vi "RoboTaxi VI_Wifi.vi"() -> ()   [LabVIEW 2022 SP3]
doc: "This example performs writes and reads on a serial port, as directed by the user. You can press the Write and Read buttons, and change the Read Count, while the example is running.\n\nThe parameters set for the serial port must match the parameters of the connected instrument or device. In this example, the Read Count parameter specifies the number of bytes that the serial port reads. If there were more bytes at the port than the specified number, those bytes would not be read. If there were less bytes at the port than the specified number, you would receive a timeout error.\n\nThis example expands upon the flow control options for XON and XOFF, allowing the user to choose those control characters. Also, the user can enable or disable a termination character. Some devices require a termination character in order to identify the end of command strings. Some devices send a termination character to signify the end of data to be read. This example shows how you can end the Read operation once a termination character is detected in the buffer and/or append a termination character at the end of the Write data."
uses:
  ESP32-PSOC-State Machine.ctl
panel:
  in  "address":string="10.0.0.127"
  in  "Stop Driving":bool
  in  "Right":bool
  in  "Left":bool
  in  "Backward":bool
  in  "Forward":bool
  in  "Manual":bool
  in  "Autonomous":bool
  in  "Track 2":bool
  in  "Track 1":bool
  out "error":bool
  out "Response 2":string
  in  "Toggle LED":bool
  in  "Enum":T1
  in  "Stop":bool
  out "Read Count":u32=1000
  out "Response":string
  # "ESP32 Control"
  # "Track Selection"
  # "Driving Mode"
  # "Manual Override"
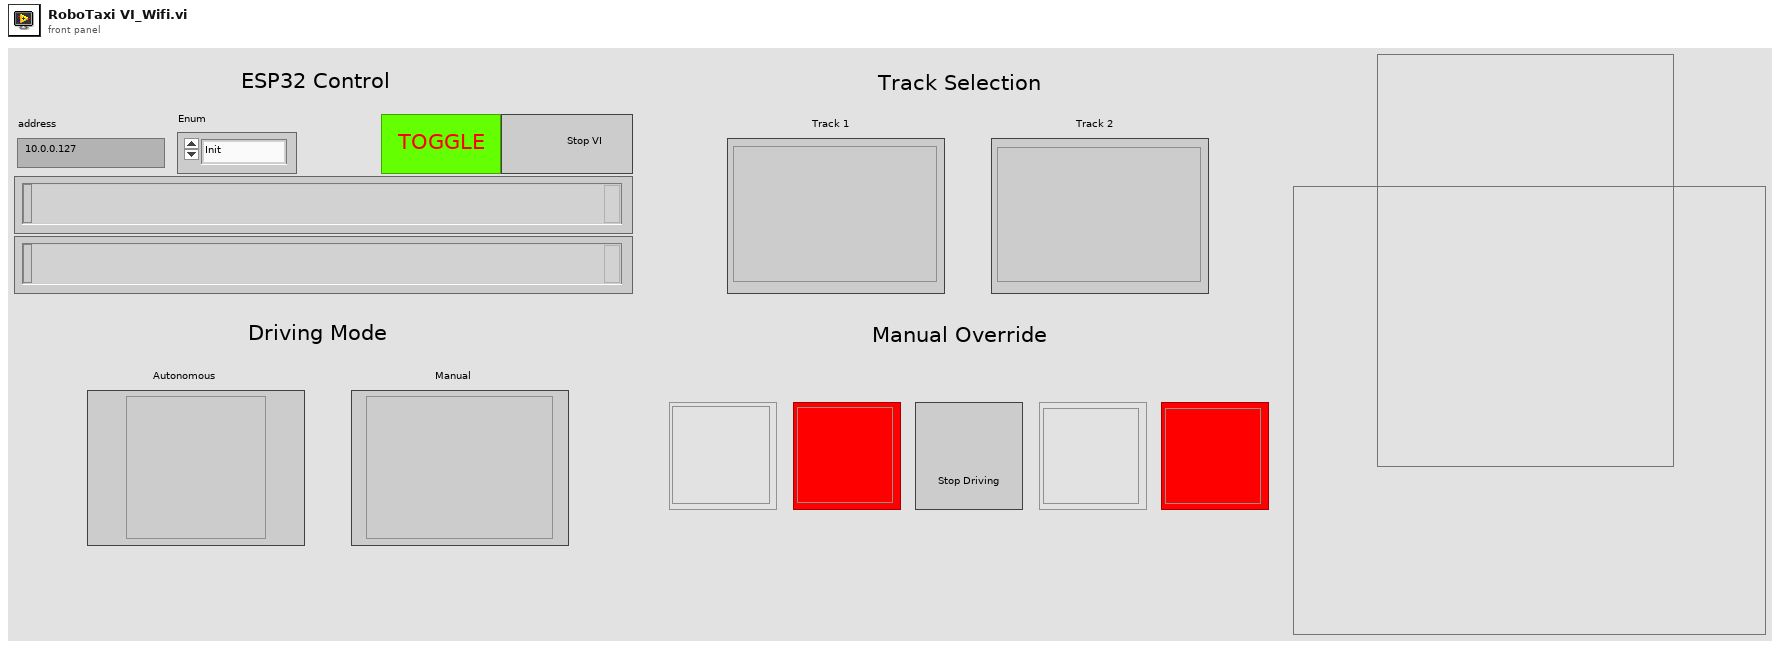
[diagram p1: front panel]
types:
  T1 = typedef "ESP32-PSOC-State Machine.ctl" = enum8{"Init", "Connect", "idle", "send", "wait", "receive", "que", "error", "exit"}
  T2 = enum16{"Standard", "Buffered", "CRLF", "Immediate"}
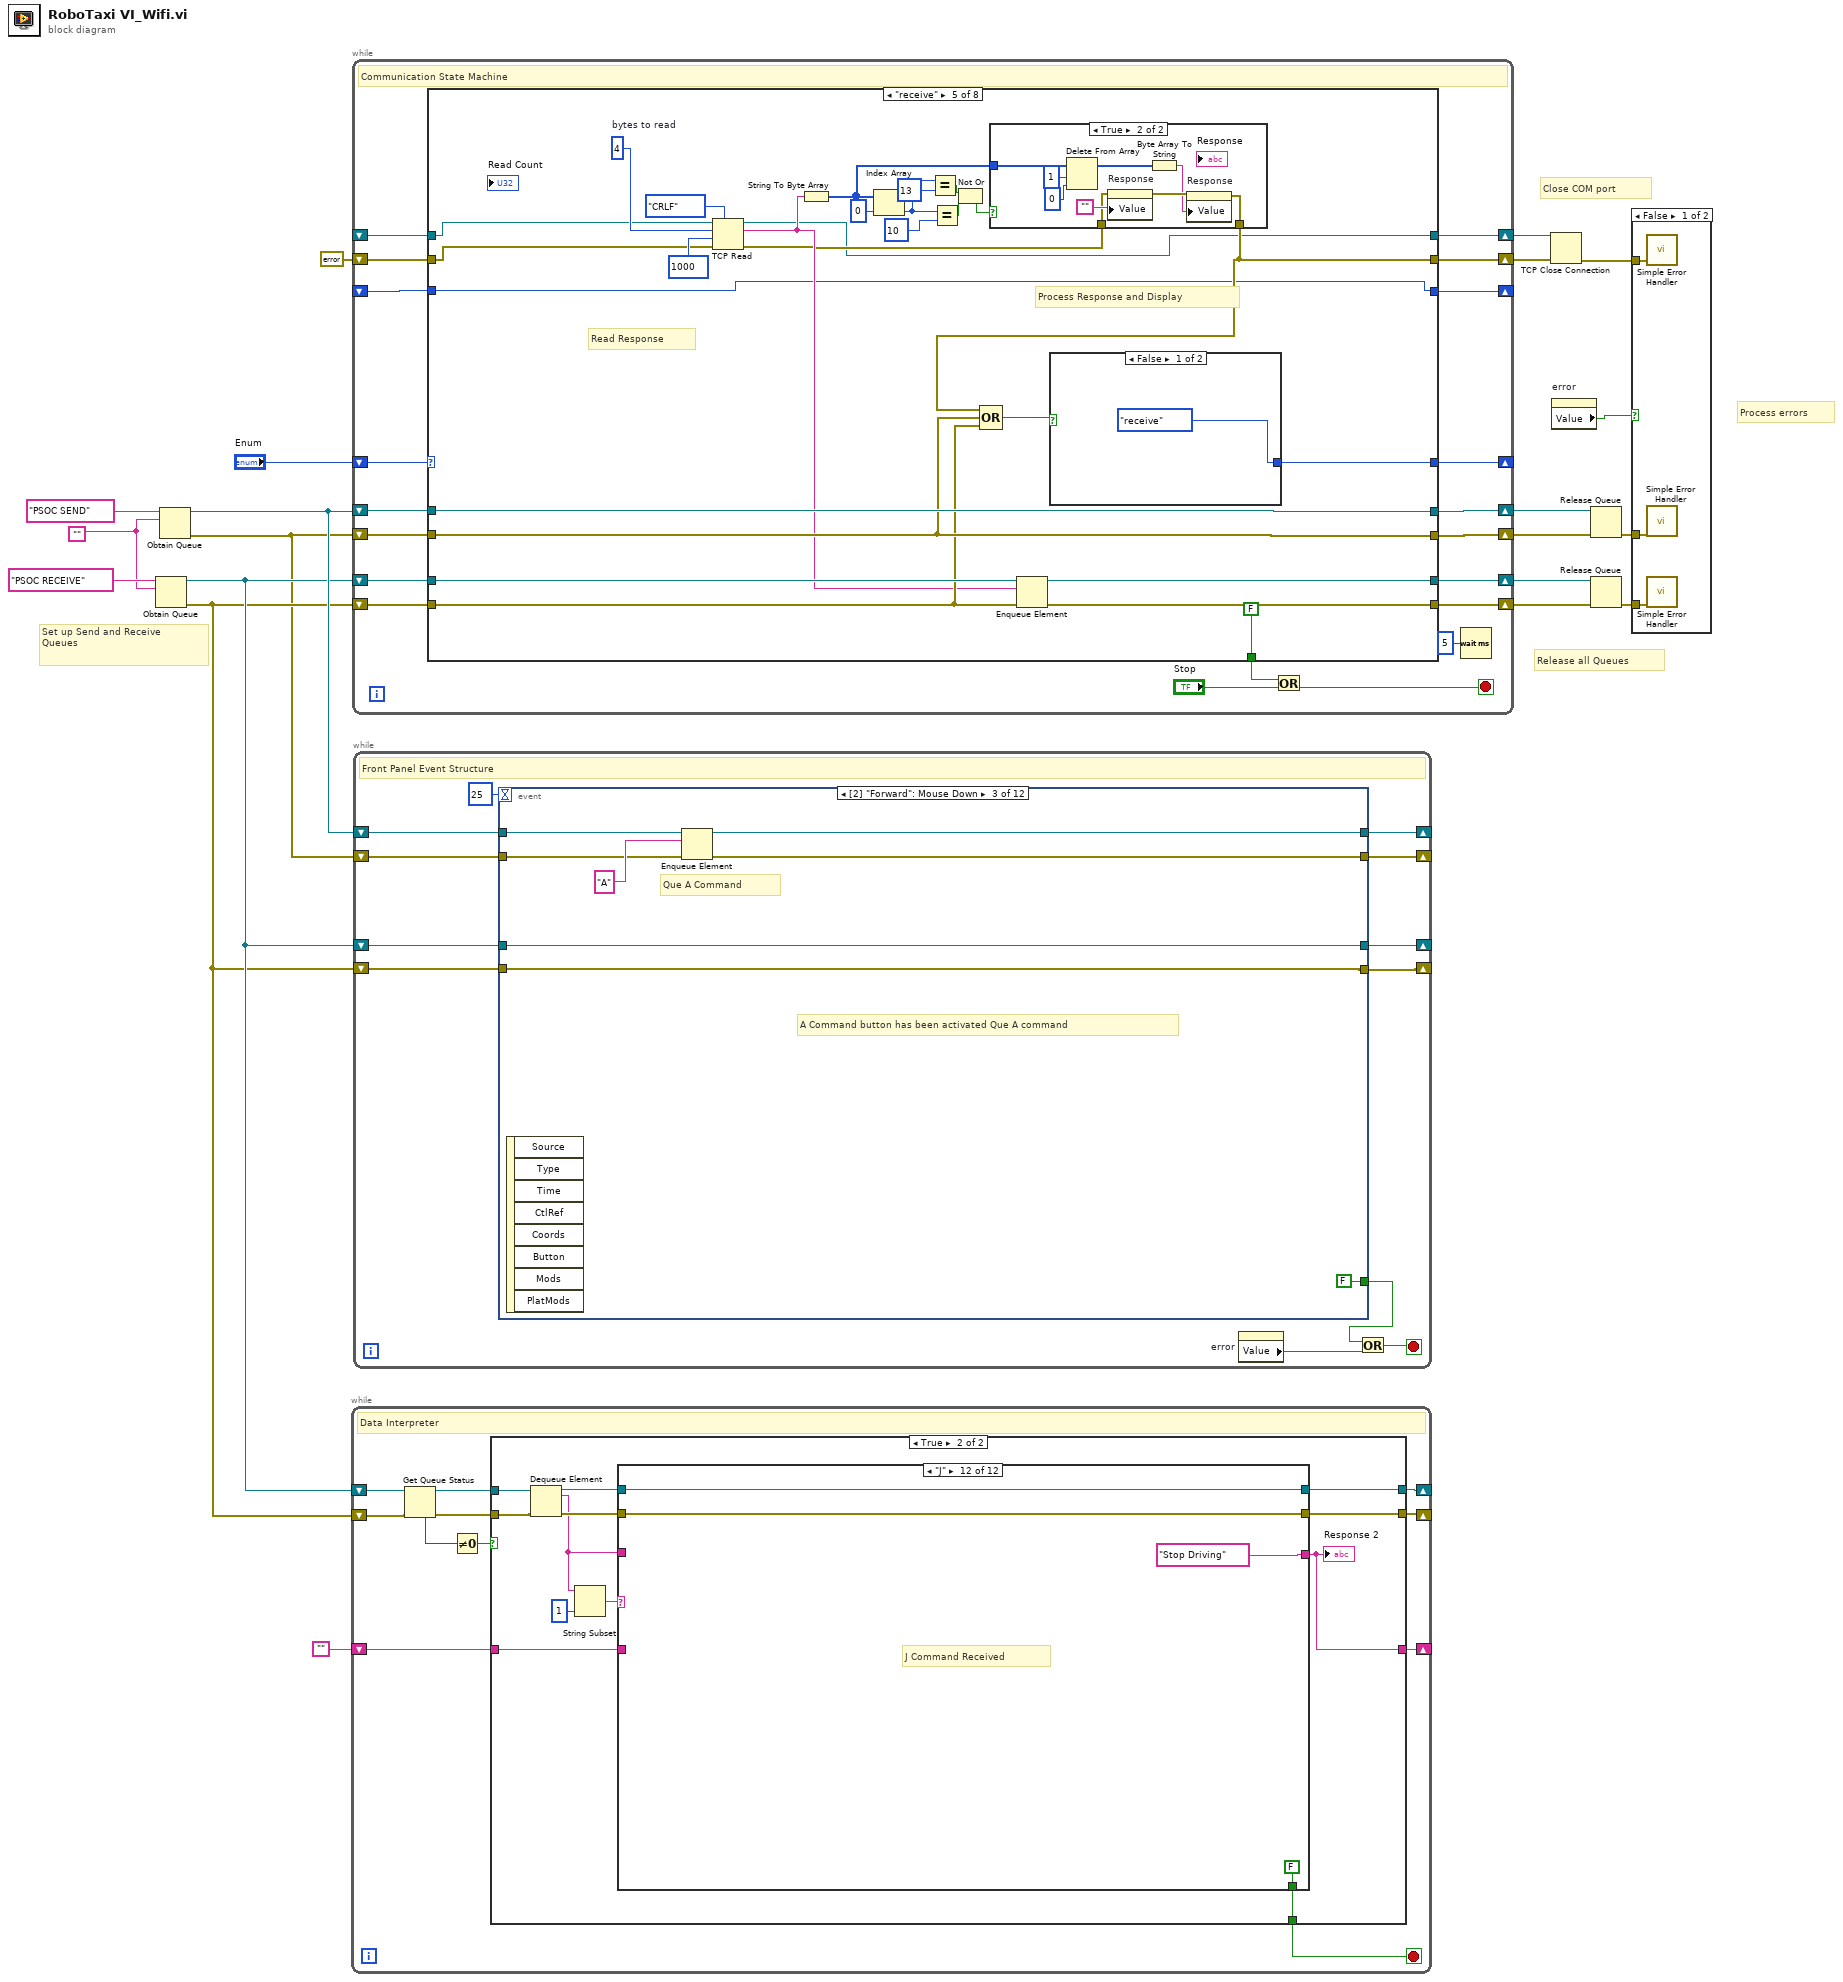
[diagram p0: block diagram]
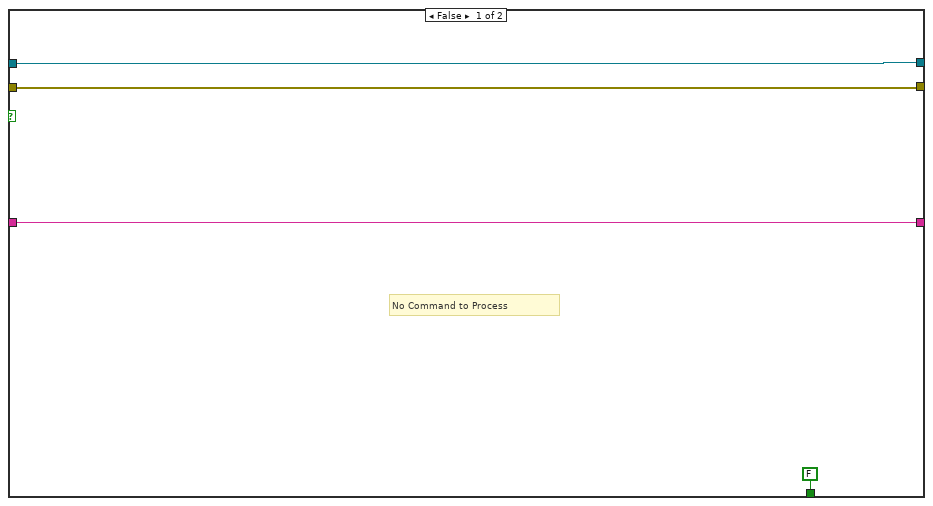
[diagram p3: hidden frame]
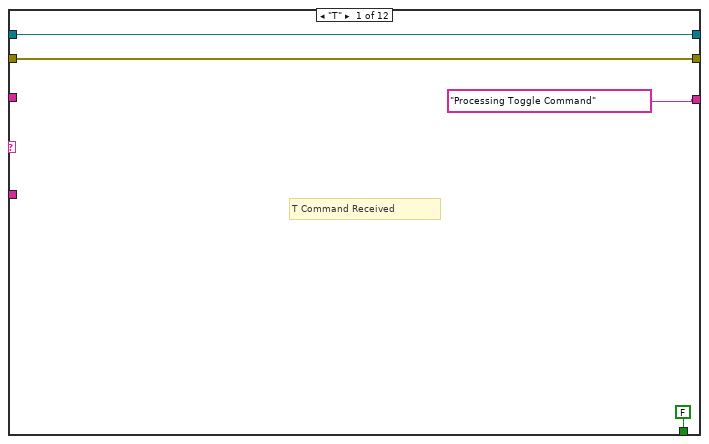
[diagram p4: hidden frame]
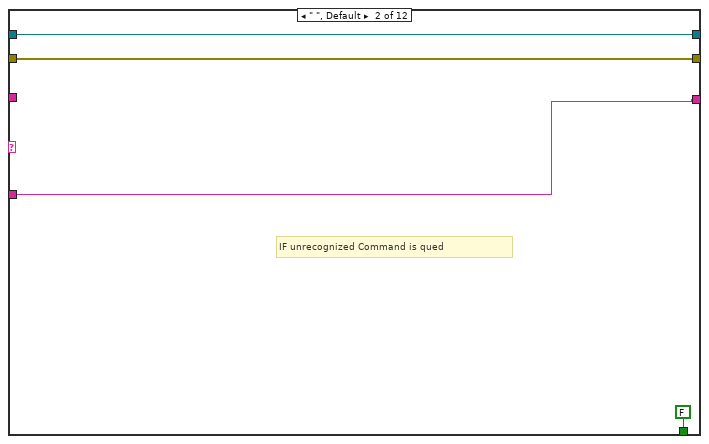
[diagram p5: hidden frame]
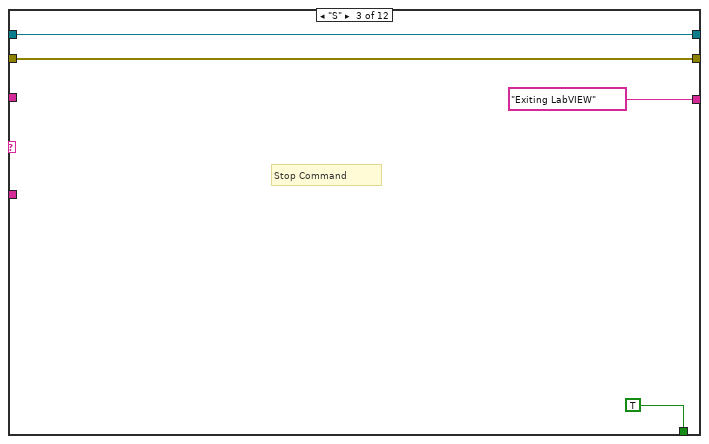
[diagram p6: hidden frame]
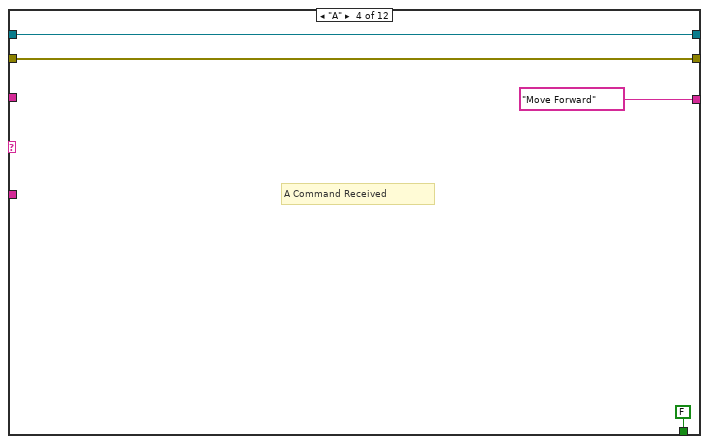
[diagram p7: hidden frame]
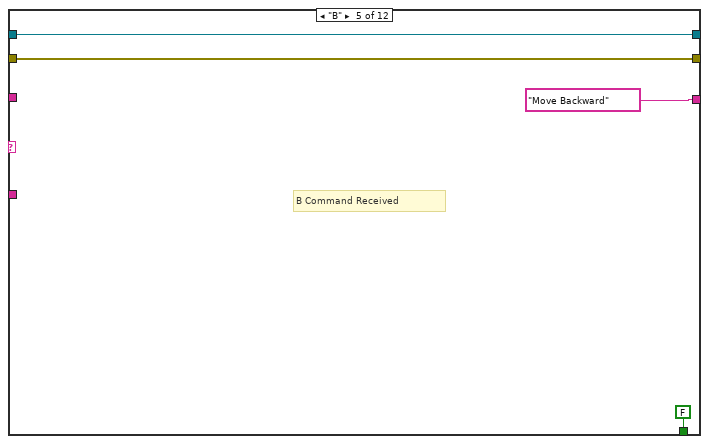
[diagram p8: hidden frame]
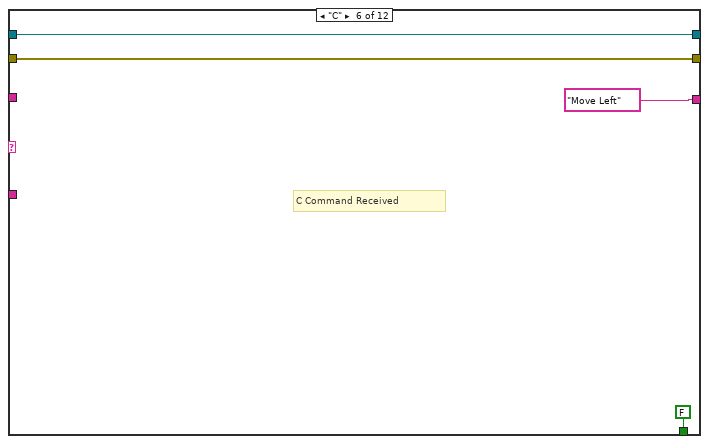
[diagram p9: hidden frame]
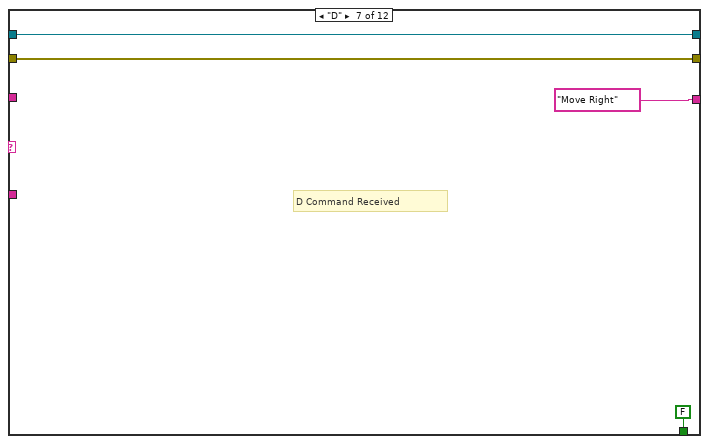
[diagram p10: hidden frame]
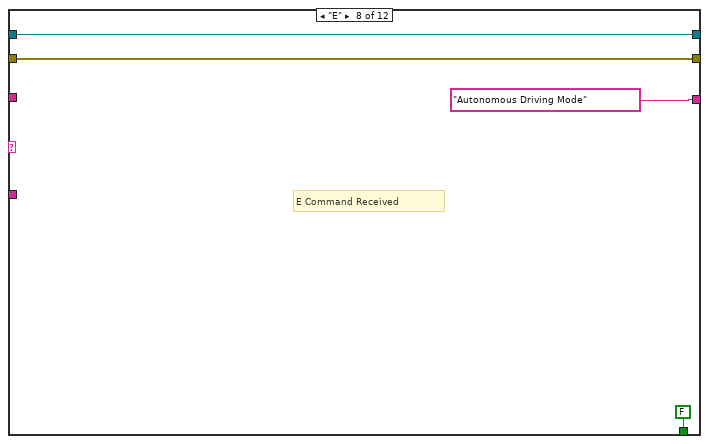
[diagram p11: hidden frame]
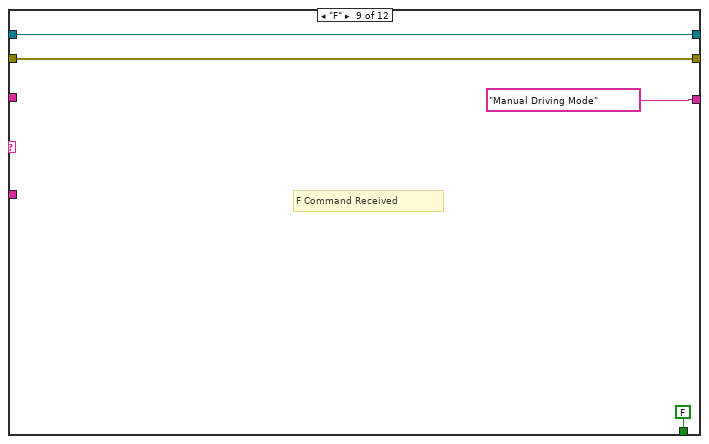
[diagram p12: hidden frame]
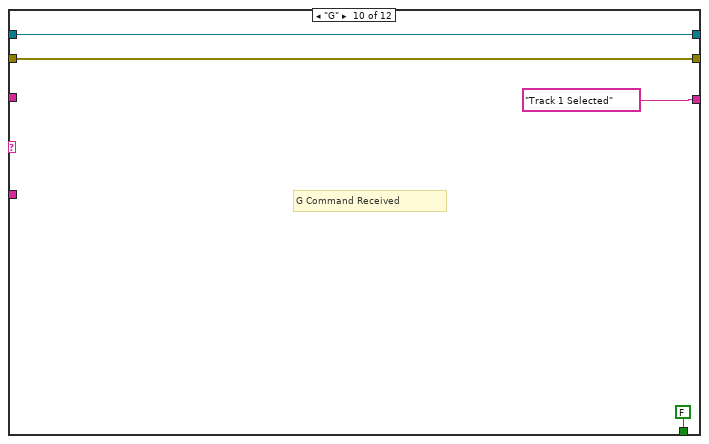
[diagram p13: hidden frame]
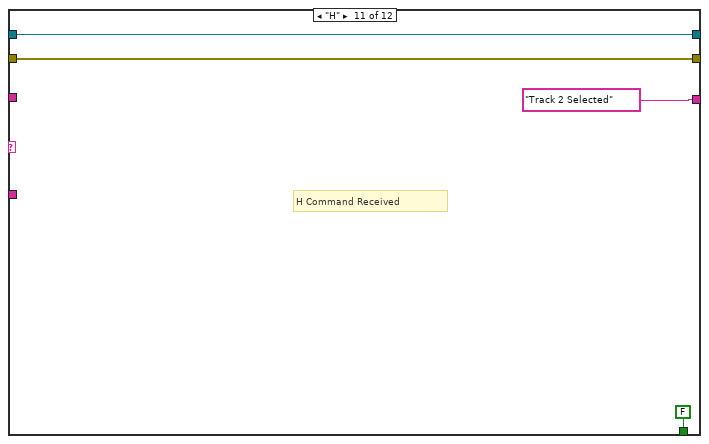
[diagram p14: hidden frame]
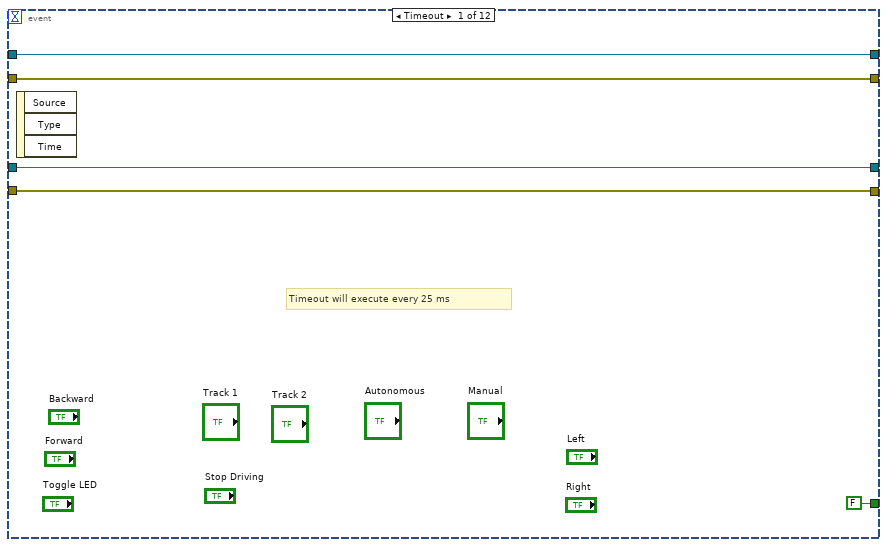
[diagram p15: hidden frame]
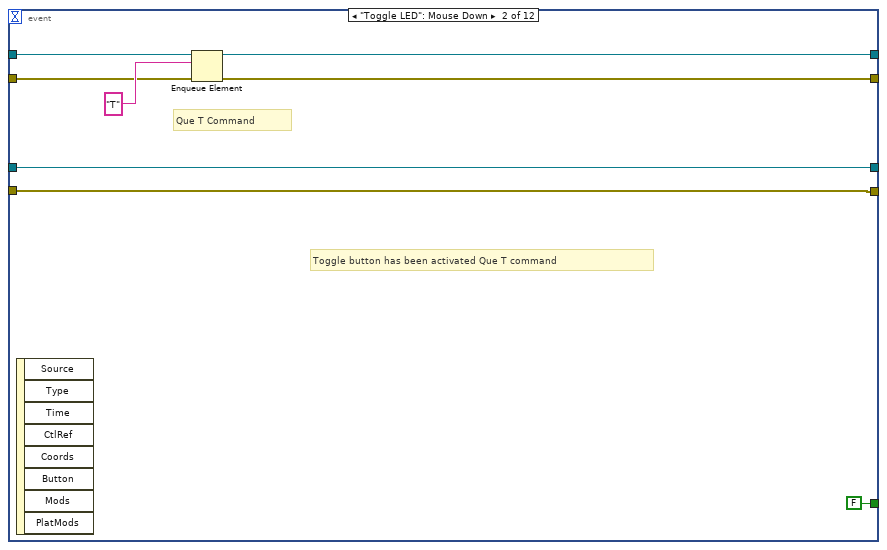
[diagram p16: hidden frame]
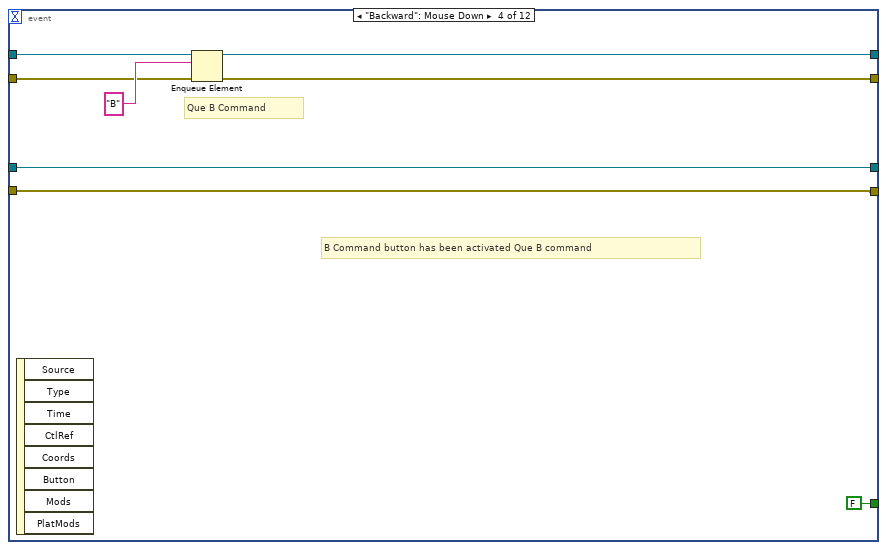
[diagram p17: hidden frame]
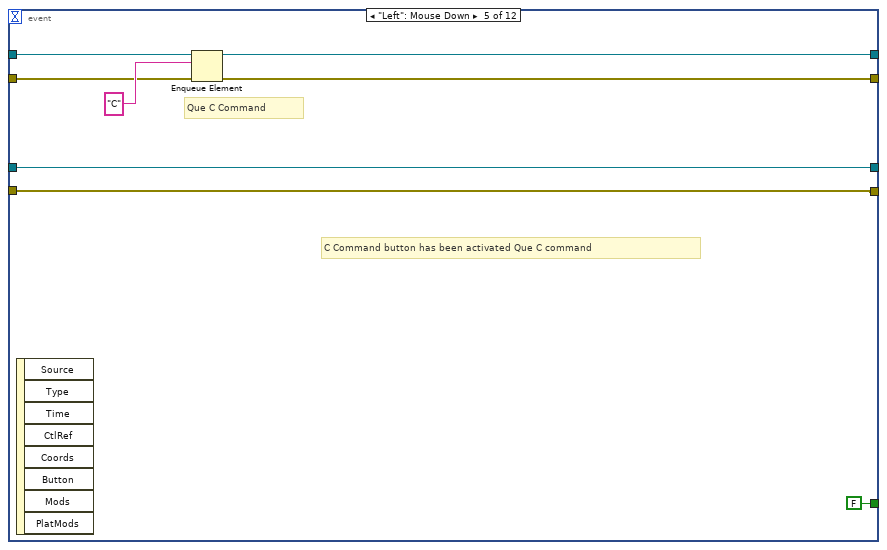
[diagram p18: hidden frame]
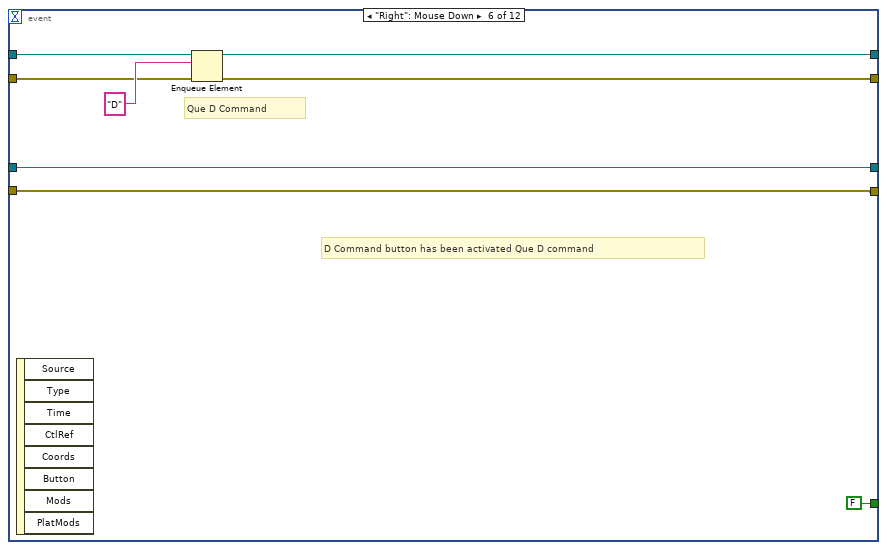
[diagram p19: hidden frame]
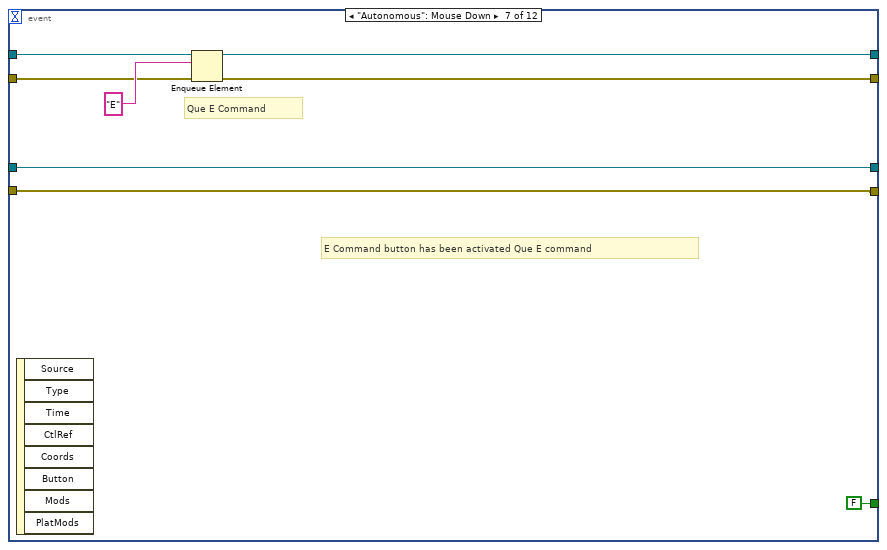
[diagram p20: hidden frame]
diagram:
  w12 = ""
  # "Process errors"
  # "Release all Queues"
  # "Close COM port"
  # "Set up Send and Receive\nQueues"
  n1 = Obtain Queue(name (unnamed)="PSOC RECEIVE", element data type=w12) -> (queue out=w11:refnum<queue>, error out=w10:errorcluster)  [unwired: 3 in, 1 out]
  n2 = Obtain Queue(name (unnamed)="PSOC SEND", element data type=w12) -> (queue out=w14:refnum<queue>, error out=w5:errorcluster)  [unwired: 3 in, 1 out]
  n3 = while {
    shift-right: [w25] -> _
    shift-left: w11 -> [w31]
    shift-right: [w24] -> _
    shift-left: w10 -> [w30]
    shift-right: [w22] -> _
    shift-left: "" -> [w21]
    stop <- w23 stop-if-true
    # "Data Interpreter"
    n4 = Get Queue Status(queue=w31, error in (no error)=w30) -> (queue out=w27:refnum<queue>, error out=w26:errorcluster, # elements in queue=w29:i32)  [unwired: 1 in, 5 out]
    n5 = Not Equal To 0?(x=w29) -> (x != 0?=w28:bool)
    n6 = case shown="True" w28 {
      tunnel: w27 -> [w35 w47]
      tunnel: w26 -> [w34 w46]
      tunnel: [w35 w41] -> w25
      tunnel: [w34 w40] -> w24
      tunnel: [FALSE w39] -> w23
      tunnel: [w32 w37] -> w22
      tunnel: w21 -> [w32 w36]
      frame False {
        # "No Command to Process"
      }
      frame True {
        n7 = Dequeue Element(queue=w47, error in (no error)=w46) -> (queue out=w45:refnum<queue>, element=w38:string, error out=w44:errorcluster)  [unwired: 1 in, 1 out]
        n8 = String Subset(string=w38, length (rest)=1 ("length (rest)")) -> (substring=w42:string)  [unwired: 1 in]
        n9 = case shown="\"J\"" w42 {
          tunnel: w45 -> [w51 w55 w59 w63 w67 w71 w75 w79 w83 w87 w91 w95]
          tunnel: w44 -> [w50 w54 w58 w62 w66 w70 w74 w78 w82 w86 w90 w94]
          tunnel: [w51 w55 w59 w63 w67 w71 w75 w79 w83 w87 w91 w95] -> w41
          tunnel: [w50 w54 w58 w62 w66 w70 w74 w78 w82 w86 w90 w94] -> w40
          tunnel: w38 -> [_ _ _ _ _ _ _ _ _ _ _ _]
          tunnel: [FALSE FALSE TRUE FALSE FALSE FALSE FALSE FALSE FALSE FALSE FALSE FALSE] -> w39
          tunnel: ["Processing Toggle Command" w52 "Exiting LabVIEW" "Move Forward" "Move Backward" "Move Left" "Move Right" "Autonomous Driving Mode" "Manual Driving Mode" "Track 1 Selected" "Track 2 Selected" "Stop Driving"] -> w37
          tunnel: w36 -> [_ w52 _ _ _ _ _ _ _ _ _ _]
          frame "T" {
            # "T Command Received"
          }
          frame " ", Default {
            # "IF unrecognized Command is qued"
          }
          frame "S" {
            # "Stop Command"
          }
          frame "A" {
            # "A Command Received"
          }
          frame "B" {
            # "B Command Received"
          }
          frame "C" {
            # "C Command Received"
          }
          frame "D" {
            # "D Command Received"
          }
          frame "E" {
            # "E Command Received"
          }
          frame "F" {
            # "F Command Received"
          }
          frame "G" {
            # "G Command Received"
          }
          frame "H" {
            # "H Command Received"
          }
          frame "J" {
            # "J Command Received"
          }
        }
        "Response 2" <- w37
      }
    }
  }
  n10 = while {
    shift-right: [w107] -> w20
    shift-left: w14 -> [w115]
    shift-right: [w106] -> w18
    shift-left: w5 -> [w114]
    shift-right: [w105] -> w19
    shift-left: w11 -> [w113]
    shift-right: [w104] -> w15
    shift-left: w10 -> [w112]
    shift-right: [w99] -> _
    shift-left: "Enum" -> [w98]
    shift-right: [w111] -> w3
    shift-left: _ -> [w108]
    shift-right: [w110] -> w2
    shift-left: errorcluster {"status"=FALSE, "code"=0, "source"=""} ("error out") -> [w109]
    shift-right: [w103] -> _
    shift-left: _ -> [w102]
    stop <- w97 stop-if-true
    # "Communication State Machine"
    n11 = case shown="\"receive\"" w98 {
      selector: w98 -> [_ _ _ _ _ _ w263 _]
      tunnel: [w128 w145 w181 w197 w228 w250 w262 w286] -> w107
      tunnel: [w123 w137 w177 w194 w220 w247 w261 w285] -> w106
      tunnel: [w126 w143 w178 w198 w229 ESP32-PSOC-State_Machine."exit" ("Enum") w263 ESP32-PSOC-State_Machine."idle" ("Enum")] -> w99
      tunnel: w115 -> [w128 w147 w183 w197 w228 w250 w262 w286]
      tunnel: w114 -> [w123 w146 w182 w194 w220 w247 w261 w285]
      tunnel: w113 -> [w129 w141 w180 w196 w227 w249 w260 w284]
      tunnel: w112 -> [w122 w136 w176 w193 w219 w246 w254 w283]
      tunnel: [w117 w133 w168 w190 w204 w252 w266 w269] -> w111
      tunnel: [w116 w132 w161 w189 w221 w248 w265 w268] -> w110
      tunnel: w109 -> [w118 w138 w166 w189 w206 w248 w265 w276]
      tunnel: w108 -> [_ w139 w165 w191 w207 w252 w266 w277]
      tunnel: [w129 w141 w180 w196 w225 w249 w258 w284] -> w105
      tunnel: [w122 w136 w176 w193 w226 w246 w256 w283] -> w104
      tunnel: [u32 0 ("Bytes at Port") w140 w179 w188 w203 w251 w264 w267] -> w103
      tunnel: w102 -> [_ w140 w179 w188 w203 w251 w264 w267]
      tunnel: [FALSE FALSE FALSE FALSE FALSE FALSE TRUE FALSE] -> w96
      frame "Init", Default {
        w120 = u16 80  # port
        # "Init State ::  Set up Serial COM port"
        n12 = TCP Open Connection(address="address", remote port or service name=w120, error in (no error)=w118) -> (connection ID=w117:refnum<k5>, error out=w116:errorcluster)  [unwired: 2 in]
        n13 = Or(x=w122, y=w123) -> (x .or. y?=w124:bool)
        n14 = Or(x=w116, y=w124) -> (x .or. y?=w125:bool)
        n15 = case shown="False" w125 {
          tunnel: [ESP32-PSOC-State_Machine."Connect" ("Enum") ESP32-PSOC-State_Machine."error" ("Enum")] -> w126
          frame False {
          }
          frame True {
          }
        }
      }
      frame "idle" {
        # "Wait until Command is in queue"
        n16 = Get Queue Status(queue=w147, error in (no error)=w146) -> (queue out=w145:refnum<queue>, error out=w137:errorcluster, # elements in queue=w144:i32)  [unwired: 1 in, 5 out]
        n17 = Not Equal To 0?(x=w144) -> (x != 0?=w142:bool)
        n18 = while {
          tunnel: w139 -> [w156]
          tunnel: w138 -> [w157]
          tunnel: [w158] -> w132
          tunnel: [w155] -> w133
          stop <- w154 continue-if-true
          w153 = 4  # bytes to read
          # "Clear Boot Message"
          n19 = TCP Read(connection ID=w156, bytes to read=w153, error in (no error)=w157, 7:T2."CRLF" ("mode (standard)"), 9:1000 ("timeout ms (25000)")) -> (connection ID out=w155:refnum<k5>, error out=w158:errorcluster)  [unwired: 1 out]
          n20 = Not Equal To 0?(x=w153) -> (x != 0?=w154:bool)
        }
        n21 = Compound Arithmetic op=OR(w132, w137, w136) -> (w135:bool)
        n22 = case shown="True" w135 {
          tunnel: [w149 ESP32-PSOC-State_Machine."error" ("Enum")] -> w143
          tunnel: w142 -> [w148 _]
          frame False {
            n23 = case shown="False" w148 {
              tunnel: [ESP32-PSOC-State_Machine."idle" ("Enum") ESP32-PSOC-State_Machine."send" ("Enum")] -> w149
              frame False {
              }
              frame True {
              }
            }
          }
          frame True {
          }
        }
      }
      frame "send" {
        w169 = 4  # bytes to read
        # "Read and Discard Echo Command"
        # "Wait for Response"
        # "Send Command"
        n24 = Dequeue Element(queue=w183, error in (no error)=w182) -> (queue out=w181:refnum<queue>, element=w172:string, error out=w177:errorcluster)  [unwired: 1 in, 1 out]
        n25 = Concatenate Strings(w172, "\r\n") -> (w167:string)
        n26 = TCP Write(connection ID=w165, data in=w167, error in (no error)=w166) -> (connection ID out=w164:refnum<k5>, error out=w162:errorcluster)  [unwired: 1 in, 1 out]
        n27 = flat-sequence {
          tunnel: [w184] -> w163
          tunnel: w164 -> [w184]
          frame #0 {
            n28 = Wait (ms)(milliseconds to wait=u32 15) -> ()  [unwired: 1 out]
          }
        }
        n29 = TCP Read(connection ID=w163, bytes to read=w169, error in (no error)=w162, 7:T2."CRLF" ("mode (standard)"), 9:1000 ("timeout ms (25000)")) -> (connection ID out=w168:refnum<k5>, error out=w161:errorcluster)  [unwired: 1 out]
        n30 = Compound Arithmetic op=OR(w161, w177, w176) -> (w175:bool)
        n31 = case shown="False" w175 {
          tunnel: [ESP32-PSOC-State_Machine."wait" ("Enum") ESP32-PSOC-State_Machine."error" ("Enum")] -> w178
          frame False {
          }
          frame True {
          }
        }
      }
      frame "wait" {
        # "Wait for actual Response"
        n32 = flat-sequence {
          tunnel: w191 -> [w200]
          tunnel: [w200] -> w190
          frame #0 {
            n33 = Wait (ms)(milliseconds to wait=u32 15) -> ()  [unwired: 1 out]
          }
        }
        n34 = Compound Arithmetic op=OR(w189, w194, w193) -> (w195:bool)
        n35 = case shown="False" w195 {
          tunnel: [ESP32-PSOC-State_Machine."receive" ("Enum") ESP32-PSOC-State_Machine."error" ("Enum")] -> w198
          frame False {
          }
          frame True {
          }
        }
      }
      frame "receive" {
        w209 = 4  # bytes to read
        # "Process Response and Display"
        # "Read Response"
        n36 = TCP Read(connection ID=w207, bytes to read=w209, error in (no error)=w206, 7:T2."CRLF" ("mode (standard)"), 9:1000 ("timeout ms (25000)")) -> (connection ID out=w204:refnum<k5>, data out=w208:string, error out=w205:errorcluster)
        n37 = String To Byte Array(string=w208) -> (unsigned byte array=w222:u8[])
        n38 = Index Array(array=w222, index=0) -> (element=w216:u8)
        n39 = Equal?(x=w216, y=u8 13) -> (x = y?=w214:bool)
        n40 = Equal?(x=w216, y=u8 10) -> (x = y?=w213:bool)
        n41 = Not Or(1:w213, 2:w214) -> (0:w212:bool)
        n42 = case shown="True" w212 {
          tunnel: w222 -> [_ w241]
          tunnel: [w232 w234] -> w221
          tunnel: w205 -> [w232 w233]
          frame False {
          }
          frame True {
            n43 = Delete From Array(array=w241, length=1, index=0) -> (array with subset deleted=w238:u8[])  [unwired: 1 out]
            n44 = property on="Response" class="Str"(error in=w233, "Value"="") -> (error out=w236:errorcluster)  [unwired: 1 in, 1 out]
            n45 = Byte Array To String(unsigned byte array=w238) -> (string=w235:string)
            n46 = property on="Response" class="Str"(error in=w236, "Value"=w235) -> (error out=w234:errorcluster)  [unwired: 1 in, 1 out]
          }
        }
        n47 = Compound Arithmetic op=OR(w221, w220, w219) -> (w218:bool)
        n48 = Enqueue Element(queue=w227, element=w208, error in (no error)=w219) -> (queue out=w225:refnum<queue>, error out=w226:errorcluster)  [unwired: 1 in, 1 out]
        n49 = case shown="False" w218 {
          tunnel: [ESP32-PSOC-State_Machine."receive" ("Enum") ESP32-PSOC-State_Machine."error" ("Enum")] -> w229
          frame False {
          }
          frame True {
          }
        }
      }
      frame "error" {
        # "Process any error"
        n50 = Build Array(w248, w247, w246) -> (w245:errorcluster[])
        n51 = for {
          tunnel: w245 -> [w253] mode=indexing
          n52 = call <vilib>:"General Error Handler.vi"("error in (no error)"=w253) -> ()  [unwired: 10 in, 5 out]
        }
        "error" <- TRUE ("error")
      }
      frame "exit" {
        (unwired) FALSE ("Connected")
        # "Exit due to error"
        n53 = Enqueue Element(queue=w260, element="S", error in (no error)=w254) -> (queue out=w258:refnum<queue>)  [unwired: 1 in, 2 out]
        n54 = property on="Response" class="Str"("Value"="") -> (error out=w256:errorcluster)  [unwired: 2 in, 1 out]
      }
      frame "Connect" {
        w273 = 4  # bytes to read
        # "Validating connection"
        # "Send ID to validate connection"
        # "Clear any residual characters"
        n55 = Concatenate Strings("I" ("write buffer"), "\r\n") -> (w278:string)
        n56 = TCP Write(connection ID=w277, data in=w278, error in (no error)=w276) -> (connection ID out=w271:refnum<k5>, error out=w272:errorcluster)  [unwired: 1 in, 1 out]
        n57 = flat-sequence {
          tunnel: [w287] -> _
          tunnel: w271 -> [w287]
          tunnel: [w287] -> w270
          frame #0 {
            n58 = Wait (ms)(milliseconds to wait=u32 5) -> ()  [unwired: 1 out]
          }
        }
        n59 = TCP Read(connection ID=w270, bytes to read=w273, error in (no error)=w272, 7:T2."CRLF" ("mode (standard)"), 9:1000 ("timeout ms (25000)")) -> (connection ID out=w269:refnum<k5>, error out=w268:errorcluster)  [unwired: 1 out]
      }
    }
    n60 = Or(x=w96, y="Stop") -> (x .or. y?=w97:bool)
    n61 = Wait (ms)(milliseconds to wait=u32 5) -> ()  [unwired: 1 out]
  }
  n62 = while {
    shift-right: [w297] -> _
    shift-left: w14 -> [w298]
    shift-right: [w296] -> _
    shift-left: w5 -> [w299]
    shift-right: [w292] -> _
    shift-left: w11 -> [w295]
    shift-right: [w293] -> _
    shift-left: w10 -> [w294]
    stop <- w289 stop-if-true
    # "Front Panel Event Structure"
    n63 = event shown="[2] \"Forward\": Mouse Down" {
      selector: _ -> [_ _ _ _ _ _ _ _ _ _ _ _]
      dyn-events: _ -> [_ _ _ _ _ _ _ _ _ _ _ _]
      timeout: 25 -> [_ _ _ _ _ _ _ _ _ _ _ _]
      tunnel: w299 -> [w303 w311 w319 w327 w335 w343 w351 w359 w367 w375 w383 w392]
      tunnel: w298 -> [w304 w313 w321 w329 w337 w345 w353 w361 w369 w377 w385 w393]
      tunnel: [w304 w310 w318 w326 w334 w342 w350 w358 w366 w374 w382 w393] -> w297
      tunnel: [w303 w309 w317 w325 w333 w341 w349 w357 w365 w373 w381 w392] -> w296
      tunnel: [FALSE FALSE FALSE FALSE FALSE FALSE FALSE FALSE FALSE FALSE FALSE TRUE] -> w291
      tunnel: w295 -> [w302 w307 w315 w323 w331 w339 w347 w355 w363 w371 w379 w391]
      tunnel: w294 -> [w301 w306 w314 w322 w330 w338 w346 w354 w362 w370 w378 w389]
      tunnel: [w301 w306 w314 w322 w330 w338 w346 w354 w362 w370 w378 w387] -> w293
      tunnel: [w302 w307 w315 w323 w331 w339 w347 w355 w363 w371 w379 w388] -> w292
      event Timeout {
        # "Timeout will execute every 25 ms"
        n64 = event-data() -> ()  [unwired: 1 in, 3 out]
      }
      event "Toggle LED": Mouse Down {
        # "Que T Command"
        # "Toggle button has been activated Que T command"
        n65 = event-data() -> ()  [unwired: 1 in, 8 out]
        n66 = Enqueue Element(queue=w313, element="T", error in (no error)=w311) -> (queue out=w310:refnum<queue>, error out=w309:errorcluster)  [unwired: 1 in, 1 out]
      }
      event "Forward": Mouse Down {
        # "Que A Command"
        # "A Command button has been activated Que A command"
        n67 = event-data() -> ()  [unwired: 1 in, 8 out]
        n68 = Enqueue Element(queue=w321, element="A", error in (no error)=w319) -> (queue out=w318:refnum<queue>, error out=w317:errorcluster)  [unwired: 1 in, 1 out]
      }
      event "Backward": Mouse Down {
        # "Que B Command"
        # "B Command button has been activated Que B command"
        n69 = event-data() -> ()  [unwired: 1 in, 8 out]
        n70 = Enqueue Element(queue=w329, element="B", error in (no error)=w327) -> (queue out=w326:refnum<queue>, error out=w325:errorcluster)  [unwired: 1 in, 1 out]
      }
      event "Left": Mouse Down {
        # "Que C Command"
        # "C Command button has been activated Que C command"
        n71 = event-data() -> ()  [unwired: 1 in, 8 out]
        n72 = Enqueue Element(queue=w337, element="C", error in (no error)=w335) -> (queue out=w334:refnum<queue>, error out=w333:errorcluster)  [unwired: 1 in, 1 out]
      }
      event "Right": Mouse Down {
        # "Que D Command"
        # "D Command button has been activated Que D command"
        n73 = event-data() -> ()  [unwired: 1 in, 8 out]
        n74 = Enqueue Element(queue=w345, element="D", error in (no error)=w343) -> (queue out=w342:refnum<queue>, error out=w341:errorcluster)  [unwired: 1 in, 1 out]
      }
      event "Autonomous": Mouse Down {
        # "Que E Command"
        # "E Command button has been activated Que E command"
        n75 = event-data() -> ()  [unwired: 1 in, 8 out]
        n76 = Enqueue Element(queue=w353, element="E", error in (no error)=w351) -> (queue out=w350:refnum<queue>, error out=w349:errorcluster)  [unwired: 1 in, 1 out]
      }
      event "Manual": Mouse Down {
        # "Que F Command"
        # "F Command button has been activated Que F command"
        n77 = event-data() -> ()  [unwired: 1 in, 8 out]
        n78 = Enqueue Element(queue=w361, element="F", error in (no error)=w359) -> (queue out=w358:refnum<queue>, error out=w357:errorcluster)  [unwired: 1 in, 1 out]
      }
      event "Track 1": Mouse Down {
        # "Que G Command"
        # "G Command button has been activated Que G command"
        n79 = event-data() -> ()  [unwired: 1 in, 8 out]
        n80 = Enqueue Element(queue=w369, element="G", error in (no error)=w367) -> (queue out=w366:refnum<queue>, error out=w365:errorcluster)  [unwired: 1 in, 1 out]
      }
      event "Track 2": Mouse Down {
        # "Que H Command"
        # "H Command button has been activated Que H command"
        n81 = event-data() -> ()  [unwired: 1 in, 8 out]
        n82 = Enqueue Element(queue=w377, element="H", error in (no error)=w375) -> (queue out=w374:refnum<queue>, error out=w373:errorcluster)  [unwired: 1 in, 1 out]
      }
      event "Stop Driving": Mouse Down {
        # "Que J Command"
        # "J Command button has been activated Que J command"
        n83 = event-data() -> ()  [unwired: 1 in, 8 out]
        n84 = Enqueue Element(queue=w385, element="J", error in (no error)=w383) -> (queue out=w382:refnum<queue>, error out=w381:errorcluster)  [unwired: 1 in, 1 out]
      }
      event "Stop": Value Change {
        (unwired) FALSE ("Connected")
        # "Stop Application"
        n85 = event-data() -> ()  [unwired: 1 in, 6 out]
        n86 = Enqueue Element(queue=w391, element="S", error in (no error)=w389) -> (queue out=w388:refnum<queue>)  [unwired: 1 in, 2 out]
        n87 = property on="Response" class="Str"("Value"="") -> (error out=w387:errorcluster)  [unwired: 2 in, 1 out]
      }
    }
    n88 = property on="error" class="Bool (strict)"() -> ("Value"=w290:bool)  [unwired: 2 in, 2 out]
    n89 = Or(x=w291, y=w290) -> (x .or. y?=w289:bool)
  }
  n90 = TCP Close Connection(connection ID=w3, error in (no error)=w2) -> (error out=w1:errorcluster)  [unwired: 1 in, 1 out]
  n91 = property on="error" class="Bool (strict)"() -> ("Value"=w4:bool)  [unwired: 2 in, 2 out]
  n92 = Release Queue(queue=w20, error in (no error)=w18) -> (error out=w7:errorcluster)  [unwired: 1 in, 2 out]
  n93 = Release Queue(queue=w19, error in (no error)=w15) -> (error out=w6:errorcluster)  [unwired: 1 in, 2 out]
  n94 = case shown="False" w4 {
    tunnel: w7 -> [w397 _]
    tunnel: w6 -> [w396 _]
    tunnel: w1 -> [w395 _]
    frame False {
      n95 = call <vilib>:"Simple Error Handler.vi"("error in (no error)"=w395) -> ()  [unwired: 1 in, 8 out]
      n96 = call <vilib>:"Simple Error Handler.vi"("error in (no error)"=w397) -> ()  [unwired: 1 in, 8 out]
      n97 = call <vilib>:"Simple Error Handler.vi"("error in (no error)"=w396) -> ()  [unwired: 1 in, 8 out]
    }
    frame True {
    }
  }
